vi "適應性控制_單頻率追蹤_V2(電腦模擬).vi"() -> ()   [LabVIEW 2010]
panel:
  out "當下權重":dbl[](array[numeric])
  out "權重":dbl[][](array[numeric])
  in  "stop":bool
  out "當下相位":dbl
  out "當下頻率":dbl
  in  "相位間距":dbl=1.0 min=0.0 max=180.0 step=1.0
  in  "中止相位(度)":dbl=90.0 min=-180.0 max=180.0
  in  "中止頻率(Hz)":dbl=5.0 min=0.02
  in  "初始相位(度)":dbl=-90.0 min=-180.0 max=180.0
  in  "全部誤差低於多少停止":dbl=1e-05 min=0.0
  out "模擬輸入x(t)":dbl[](graph)
  in  "頻率間距":dbl=1.0 min=0.01
  out "理想與FIR輸出":dbl[][](graph)
  out "message":string=" INSTRUCTIONS:\r\rNormal Use:  When using subVIs that incorporate the error in/error out (or error I/O) structure, place this handler where you want to inform the user of an error, typically at the end of the I/O data path, as the last action of the program.  If the error in error? is ERROR, the handler creates a message describing the error and its source.  If the type of dialog = 1 (default), the message is displayed to the user, who can only acknowedge it.  If the type = 2, the user can acknowledge the message or abort execution; aborting a program with active I/O is not recommended.  If the type = 0, no message is displayed; this is used to process the error programmatically, and the error out cluster elements are wired to individual terminals for that reason.  \r\rOther Use:\n\r\nlocal testing.  To test the error code of a subVI or function that does not have the error I/O structure, you can wire its error code and a source string to the local error code and error source inputs.  If error in error? indicates no error and error code is not equal to 0, the local code and source are substituted for the error in values, and error? is set TRUE (ERROR)."
  out "誤差":dbl(graph)
  in  "理想振幅":dbl=1.0
  in  "理想直流偏移":dbl
  in  "目標相位(deg)":dbl min=-180.0 max=180.0
  in  "收斂係數":dbl=0.001
  in  "order":i32=80
  in  "初始頻率(Hz)":dbl=1.0 min=0.01
  in  "取樣頻率":dbl=1000.0 min=1.0 max=1000.0 step=1.0
  in  "模擬直流偏移":dbl
  in  "模擬振幅振幅":dbl=1.0
  # "頻率"
  # "相位"
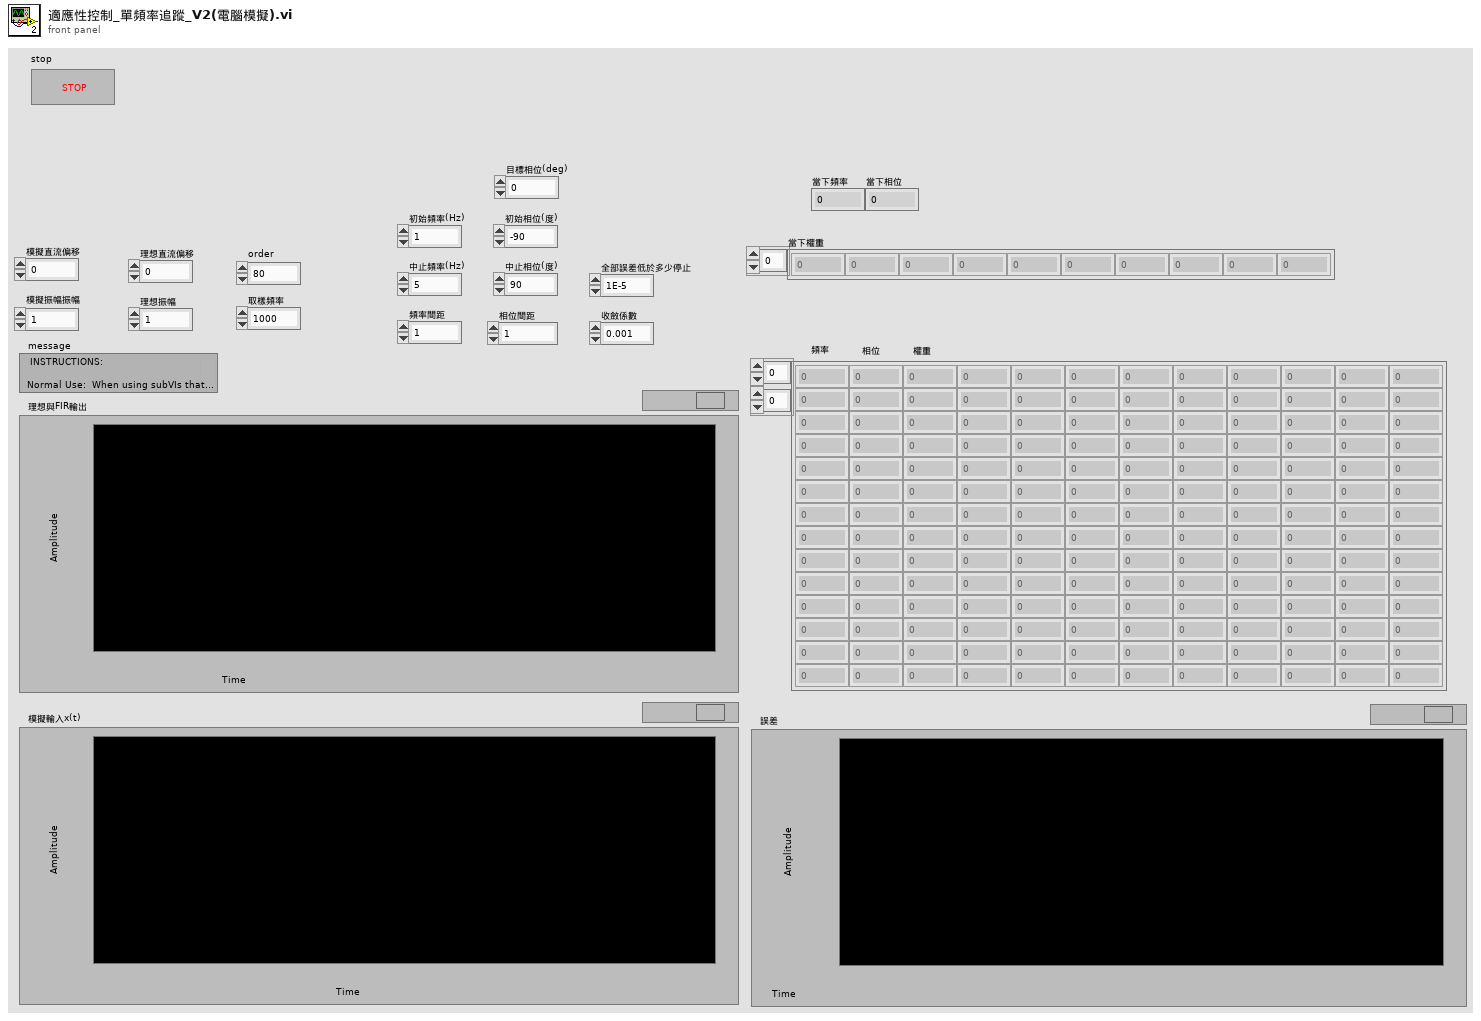
[diagram p1: front panel]
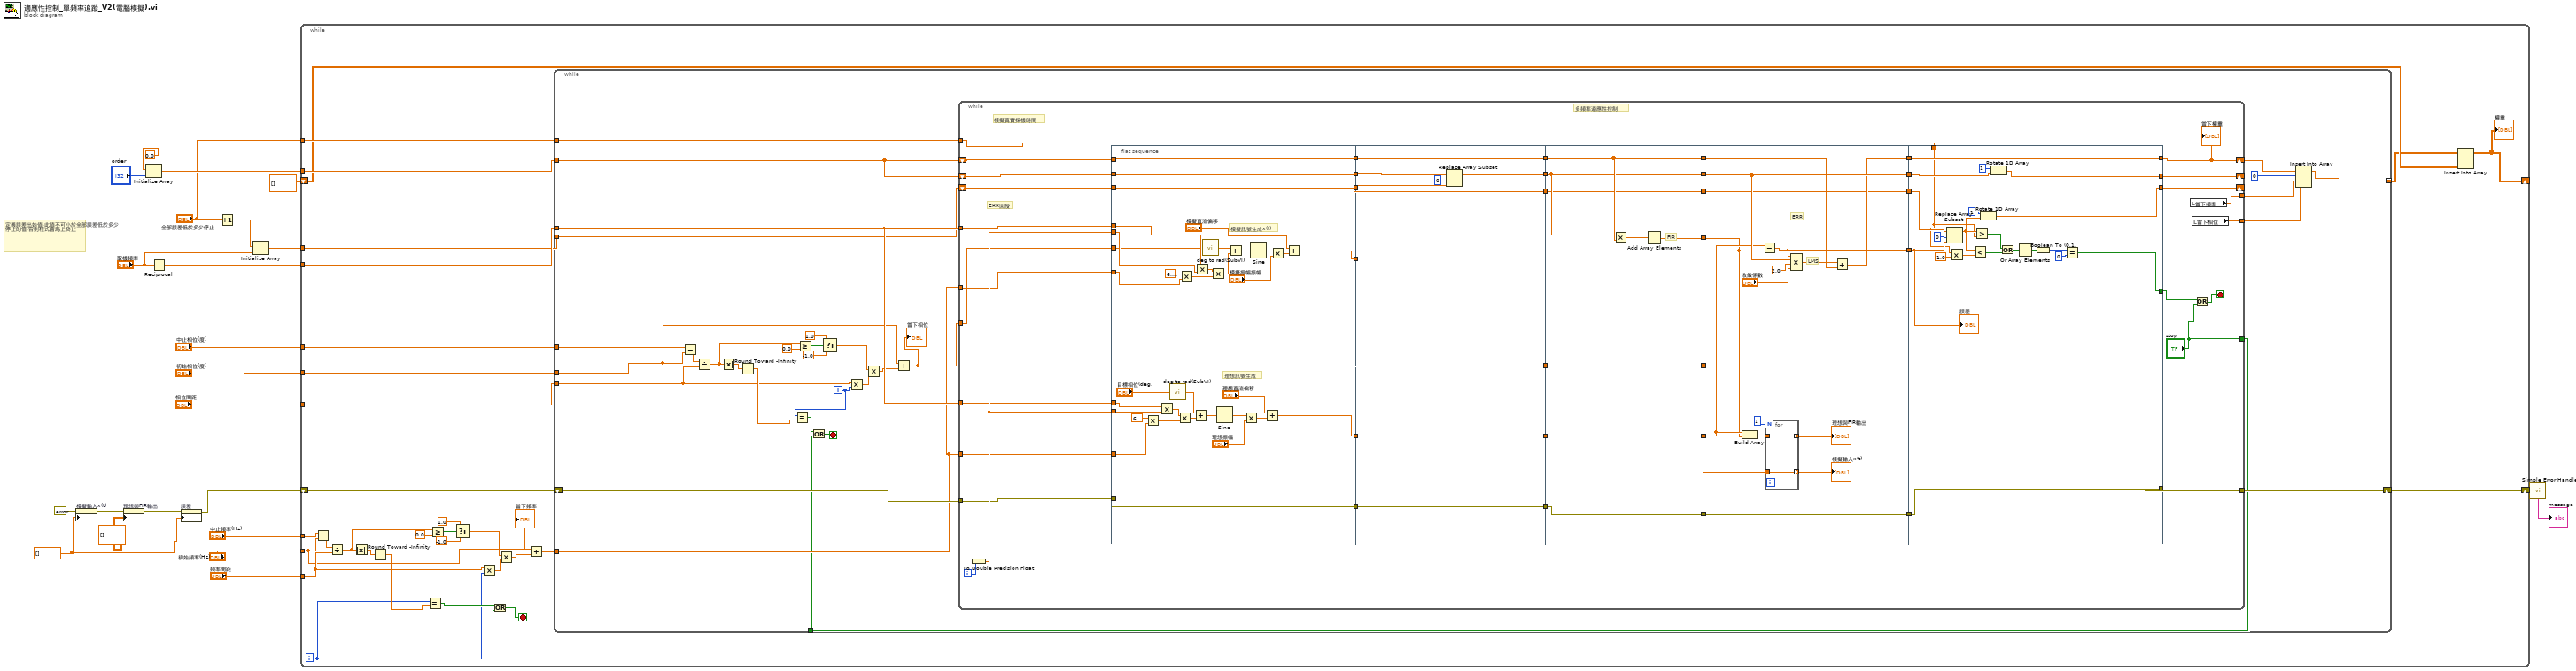
[diagram p0: block diagram]
diagram:
  w13 = dbl[] [] ("History Data")
  # "定義誤差出始值,此值不可小於全部誤差低於多少停止的值,否則程式會馬上終止"
  n1 = property on="模擬輸入x(t)" class="WFChart (strict)"(error in=errorcluster {"status"=FALSE, "code"=0, "source"=""} ("error constant"), "History Data"=w13) -> (error out=w17:errorcluster)  [unwired: 1 in, 1 out]
  n2 = property on="理想與FIR輸出" class="WFChart (strict)"(error in=w17, "History Data"=dbl[][] []) -> (error out=w18:errorcluster)  [unwired: 1 in, 1 out]
  n3 = Initialize Array(0.0 ("element"), "order") -> (w12:dbl[])
  n4 = Reciprocal(x="取樣頻率") -> (1/x=w22:dbl)
  n5 = property on="誤差" class="WFChart (strict)"(error in=w18, "History Data"=w13) -> (error out=w20:errorcluster)  [unwired: 1 in, 1 out]
  n6 = Increment(x="全部誤差低於多少停止") -> (x+1=w9:dbl)
  n7 = Initialize Array(w9, "取樣頻率") -> (w10:dbl[])
  n8 = while {
    tunnel: w22 -> [w54]
    tunnel: w12 -> [w51]
    tunnel: w10 -> [w50]
    tunnel: "全部誤差低於多少停止" -> [w49]
    tunnel: "中止相位(度)" -> [w48]
    tunnel: "初始相位(度)" -> [w47]
    tunnel: "相位間距" -> [w46]
    shift-right: [w53] -> w21
    shift-left: w20 -> [w52]
    tunnel: "中止頻率(Hz)" -> [w34]
    tunnel: "初始頻率(Hz)" -> [w32]
    tunnel: "頻率間距" -> [w33]
    shift-right: [w25] -> _
    shift-left: dbl[][] [] -> [w26]
    i -> [w27]
    stop <- w29 stop-if-true
    n9 = Subtract(x=w34, y=w32) -> (x-y=w35:dbl)
    n10 = Divide(x=w35, y=w33) -> (x/y=w36:dbl)
    n11 = Absolute Value(x=w36) -> (abs(x)=w45:dbl)
    n12 = Round Toward -Infinity(1:w45) -> (0:w44:dbl)
    n13 = Equal?(x=w27, y=w44) -> (x = y?=w30:bool)
    n14 = Greater Or Equal?(x=w36, y=0.0) -> (x >= y?=w38:bool)
    n15 = Select(t=1.0, s=w38, f=-1.0) -> (s? t:f=w40:dbl)
    n16 = Multiply(x=w33, y=w27) -> (x*y=w39:dbl)
    n17 = Multiply(x=w40, y=w39) -> (x*y=w43:dbl)
    n18 = Add(x=w32, y=w43) -> (x+y=w31:dbl)
    "當下頻率" <- w31
    n19 = while {
      tunnel: w54 -> [w85]
      tunnel: w51 -> [w82]
      tunnel: w50 -> [w81]
      tunnel: w49 -> [w80]
      shift-right: [w84] -> w53
      shift-left: w52 -> [w83]
      tunnel: w48 -> [w67]
      tunnel: w47 -> [w66]
      tunnel: w46 -> [w65]
      tunnel: w31 -> [w64]
      tunnel: [w60] -> w28
      tunnel: [w57] -> w24 mode=indexing
      i -> [w70]
      stop <- w61 stop-if-true
      n20 = Subtract(x=w67, y=w66) -> (x-y=w79:dbl)
      n21 = Divide(x=w79, y=w65) -> (x/y=w78:dbl)
      n22 = Absolute Value(x=w78) -> (abs(x)=w68:dbl)
      n23 = Round Toward -Infinity(1:w68) -> (0:w69:dbl)
      n24 = Equal?(x=w70, y=w69) -> (x = y?=w62:bool)
      n25 = Greater Or Equal?(x=w78, y=0.0) -> (x >= y?=w76:bool)
      n26 = Select(t=1.0, s=w76, f=-1.0) -> (s? t:f=w74:dbl)
      n27 = Multiply(x=w65, y=w70) -> (x*y=w75:dbl)
      n28 = Multiply(x=w74, y=w75) -> (x*y=w71:dbl)
      n29 = Add(x=w66, y=w71) -> (x+y=w63:dbl)
      "當下相位" <- w63
      n30 = while {
        shift-right: [w100] -> _
        shift-left: w82 -> [w129]
        shift-right: [w116] -> w59
        shift-left: w82 -> [w124]
        tunnel: w85 -> [w113]
        tunnel: w85 -> [w112]
        tunnel: w64 -> [w109]
        tunnel: [w108] -> w84
        tunnel: w83 -> [w103]
        tunnel: w64 -> [w99]
        shift-right: [w93] -> _
        shift-left: w81 -> [w98]
        tunnel: w80 -> [w92]
        tunnel: w63 -> [w91]
        tunnel: ["stop"] -> w60
        tunnel: [w87] -> w56
        tunnel: [w86] -> w55
        i -> [w110]
        stop <- w89 stop-if-true
        # "ERR回授"
        # "模擬真實採樣時間"
        # "多頻率適應性控制"
        n31 = To Double Precision Float(number=w110) -> (double precision float=w122:dbl)
        n32 = flat-sequence {
          tunnel: w122 -> [w164]
          tunnel: [w163] -> w130
          tunnel: w129 -> [w163]
          tunnel: [w135] -> w128
          tunnel: [w162] -> w125
          tunnel: w124 -> [w162]
          tunnel: w122 -> [w161]
          tunnel: [w146] -> w119
          tunnel: w113 -> [w160]
          tunnel: w112 -> [w159]
          tunnel: w109 -> [w133]
          tunnel: [w158] -> w104
          tunnel: w103 -> [w158]
          tunnel: w99 -> [w134]
          tunnel: w98 -> [w132]
          tunnel: [w132] -> w97
          tunnel: w91 -> [w131]
          tunnel: w130 -> [w169]
          tunnel: w128 -> [w166]
          tunnel: [w172] -> w127
          tunnel: [w171] -> w126
          tunnel: w125 -> [w171]
          tunnel: [w170] -> w120
          tunnel: w119 -> [w170]
          tunnel: [w168] -> w105
          tunnel: w104 -> [w168]
          tunnel: [w166] -> w101
          tunnel: w97 -> [w165]
          tunnel: [w165] -> w94
          tunnel: w127 -> [w174]
          tunnel: w126 -> [w180]
          tunnel: [w180] -> w123
          tunnel: [w179] -> w121
          tunnel: w120 -> [w179]
          tunnel: [w178] -> w118
          tunnel: [w174] -> w117
          tunnel: [w177] -> w106
          tunnel: w105 -> [w177]
          tunnel: [w176] -> w102
          tunnel: w101 -> [w176]
          tunnel: [w173] -> w95
          tunnel: w94 -> [w173]
          tunnel: w123 -> [w196]
          tunnel: w121 -> [w183]
          tunnel: w118 -> [w182]
          tunnel: w117 -> [w187]
          tunnel: [w184] -> w115
          tunnel: [w187] -> w114
          tunnel: [w188] -> w111
          tunnel: [w193] -> w107
          tunnel: w106 -> [w193]
          tunnel: w102 -> [w192]
          tunnel: [w181] -> w96
          tunnel: w95 -> [w181]
          tunnel: [w219] -> w116
          tunnel: w115 -> [w219]
          tunnel: w114 -> [w215]
          tunnel: [w218] -> w100
          tunnel: w111 -> [w210]
          tunnel: [w217] -> w108
          tunnel: w107 -> [w217]
          tunnel: w96 -> [w213]
          tunnel: [w211] -> w93
          tunnel: [w208] -> w90
          tunnel: w92 -> [w199]
          frame #0 {
            # "模擬訊號生成x(t)"
            # "理想訊號生成"
            n33 = Multiply(x=6.283185307179586, y=w134) -> (x*y=w155:dbl)
            n34 = Multiply(x=w159, y=w161) -> (x*y=w148:dbl)
            n35 = call "deg to rad(SubVI).vi"("Degree"="目標相位(deg)") -> ("Radian"=w152:dbl)
            n36 = Multiply(x=w148, y=w155) -> (x*y=w156:dbl)
            n37 = Multiply(x=6.283185307179586, y=w133) -> (x*y=w143:dbl)
            n38 = Add(x=w152, y=w156) -> (x+y=w157:dbl)
            n39 = Multiply(x=w160, y=w164) -> (x*y=w137:dbl)
            n40 = call "deg to rad(SubVI).vi"("Degree"=w131) -> ("Radian"=w140:dbl)
            n41 = Multiply(x=w137, y=w143) -> (x*y=w144:dbl)
            n42 = Sine(x=w157) -> (sin(x)=w153:dbl)
            n43 = Add(x=w140, y=w144) -> (x+y=w145:dbl)
            n44 = Multiply(x=w153, y="理想振幅") -> (x*y=w154:dbl)
            n45 = Sine(x=w145) -> (sin(x)=w141:dbl)
            n46 = Add(x="理想直流偏移", y=w154) -> (x+y=w146:dbl)
            n47 = Multiply(x=w141, y="模擬振幅振幅") -> (x*y=w142:dbl)
            n48 = Add(x="模擬直流偏移", y=w142) -> (x+y=w135:dbl)
          }
          frame #1 {
            n49 = Replace Array Subset(array=w169, new element=w166, index=0) -> (w172:dbl[])
          }
          frame #2 {
            # "FIR"
            n50 = Multiply(x=w174, y=w180) -> (x*y=w175:dbl[])
            n51 = Add Array Elements(numeric array=w175) -> (sum=w178:dbl)
          }
          frame #3 {
            # "LMS"
            # "ERR"
            n52 = Build Array(w183, w182) -> (w194:dbl[])
            n53 = Subtract(x=w183, y=w182) -> (x-y=w188:dbl)
            n54 = for {
              N: 1 -> [_]
              tunnel: [w198] -> w185 mode=indexing
              tunnel: w194 -> [w198]
              tunnel: [w197] -> w191 mode=indexing
              tunnel: w192 -> [w197]
            }
            "理想與FIR輸出" <- w185
            "模擬輸入x(t)" <- w191
            n55 = Compound Arithmetic op=MULTIPLY(w188, w187, 2.0, "收斂係數") -> (w186:dbl[])
            n56 = Add(x=w186, y=w196) -> (x+y=w184:dbl[])
          }
          frame #4 {
            n57 = Replace Array Subset(array=w213, new element=w210, index=0) -> (w205:dbl[])
            n58 = Multiply(x=w199, y=-1.0) -> (x*y=w207:dbl)
            n59 = Less?(x=w205, y=w207) -> (x < y?=w203:bool[])
            n60 = Greater?(x=w205, y=w199) -> (0:w204:bool[])
            n61 = Rotate 1D Array(1:w205, 2:1 ("n")) -> (0:w211:dbl[])
            n62 = Rotate 1D Array(1:w215, 2:1 ("n")) -> (0:w218:dbl[])
            n63 = Or(x=w204, y=w203) -> (x .or. y?=w202:bool[])
            n64 = Or Array Elements(Boolean array=w202) -> (logical OR=w201:bool)
            n65 = Boolean To (0,1)(Boolean=w201) -> (0, 1=w200:i16)
            n66 = Equal?(x=w200, y=u32 0) -> (x = y?=w208:bool)
            "誤差" <- w210
          }
        }
        n67 = local read "當下頻率"() -> (w86:dbl)
        n68 = local read "當下相位"() -> (w87:dbl)
        n69 = Or(x=w90, y="stop") -> (x .or. y?=w89:bool)
        "當下權重" <- w116
      }
      n70 = Or(x=w62, y=w60) -> (x .or. y?=w61:bool)
      n71 = Insert Into Array(array=w59, index=0, new element #1=w55, new element #2=w56) -> (w57:dbl[])
    }
    n72 = Or(x=w30, y=w28) -> (x .or. y?=w29:bool)
    n73 = Insert Into Array(array=w24, new element=w26) -> (w25:dbl[][])  [unwired: 2 in]
    "權重" <- w25
  }
  n74 = call <vilib>:"Simple Error Handler.vi"("error in (no error)"=w21) -> ("message"=→"message":string)  [unwired: 4 in, 4 out]
